vi "Factorial.vi"(1 "N":i32) -> (0 "N!":T1={"Array Num"=[1, 2, 3], "Decimal Index"=0, "stop"=FALSE})   [LabVIEW 2025]
uses:
  Number.ctl
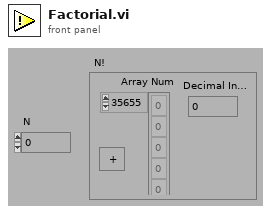
[diagram p1: front panel]
types:
  T1 = typedef "Number.ctl" = cluster{"Array Num":i8[], "Decimal Index":i32, "stop":bool}
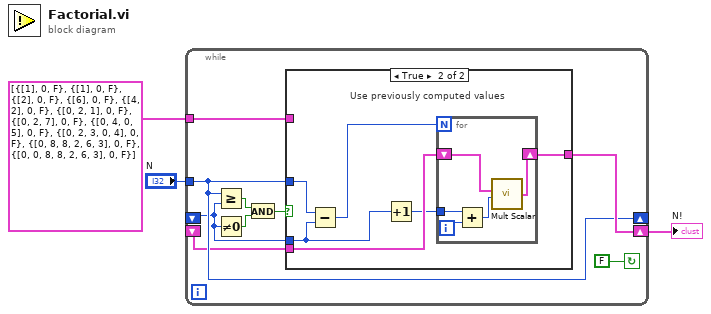
[diagram p0: block diagram]
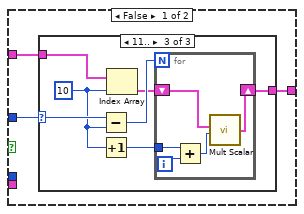
[diagram p2: hidden frame]
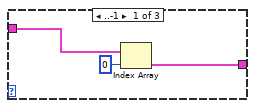
[diagram p3: hidden frame]
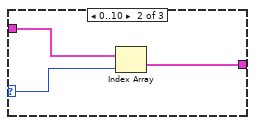
[diagram p4: hidden frame]
diagram:
  n1 = while {
    tunnel: "N" -> [w9]
    tunnel: T1[] [{"Array Num"=[1], "Decimal Index"=0, "stop"=FALSE}, {"Array Num"=[1], "Decimal Index"=0, "stop"=FALSE}, {"Array Num"=[2], "Decimal Index"=0, "stop"=FALSE}, {"Array Num"=[6], "Decimal Index"=0, "stop"=FALSE}, {"Array Num"=[4, 2], "Decimal Index"=0, "stop"=FALSE}, {"Array Num"=[0, 2, 1], "Decimal Index"=0, "stop"=FALSE}, {"Array Num"=[0, 2, 7], "Decimal Index"=0, "stop"=FALSE}, {"Array Num"=[0, 4, 0, 5], "Decimal Index"=0, "stop"=FALSE}, {"Array Num"=[0, 2, 3, 0, 4], "Decimal Index"=0, "stop"=FALSE}, {"Array Num"=[0, 8, 8, 2, 6, 3], "Decimal Index"=0, "stop"=FALSE}, {"Array Num"=[0, 0, 8, 8, 2, 6, 3], "Decimal Index"=0, "stop"=FALSE}] -> [w12]
    shift-right: [w9] -> _
    shift-left: _ -> [w7]
    shift-right: [w10] -> w1
    shift-left: _ -> [w8]
    stop <- FALSE continue-if-true
    n2 = Greater Or Equal?(x=w9, y=w7) -> (x >= y?=w5:bool)
    n3 = Not Equal To 0?(x=w7) -> (x != 0?=w4:bool)
    n4 = And(x=w5, y=w4) -> (x .and. y?=w6:bool)
    n5 = case shown="True" w6 {
      tunnel: w12 -> [w15 _]
      tunnel: [w14 w38] -> w10
      tunnel: w9 -> [w13 w37]
      tunnel: w8 -> [_ w39]
      tunnel: w7 -> [_ w35]
      frame False {
        n6 = case shown="11.." w13 {
          selector: w13 -> [_ w20 w28]
          tunnel: w15 -> [w18 w21 w26]
          tunnel: [w16 w19 w22] -> w14
          frame ..-1 {
            n7 = Index Array(array=w18, index=0) -> (element=w16:T1)
          }
          frame 0..10 {
            n8 = Index Array(array=w21, index=w20) -> (element=w19:T1)
          }
          frame 11.. {
            w24 = 10 ("index")
            n9 = Subtract(x=w28, y=w24) -> (x-y=w27:i32)
            n10 = Increment(x=w24) -> (x+1=w23:i32)
            n11 = Index Array(array=w26, index=w24) -> (element=w25:T1)
            n12 = for {
              N: w27 -> [_]
              tunnel: w23 -> [w33]
              shift-right: [w31] -> w22
              shift-left: w25 -> [w30]
              i -> [w32]
              n13 = Add(x=w33, y=w32) -> (x+y=w29:i32)
              n14 = call "Mult Scalar.vi"("A"=w30, "Scalar"=w29) -> ("A x Scalar"=w31:T1)  [unwired: 3 in]
            }
          }
        }
      }
      frame True {
        # "Use previously computed values"
        n15 = Subtract(x=w37, y=w35) -> (x-y=w36:i32)
        n16 = Increment(x=w35) -> (x+1=w34:i32)
        n17 = for {
          N: w36 -> [_]
          tunnel: w34 -> [w44]
          shift-right: [w42] -> w38
          shift-left: w39 -> [w41]
          i -> [w43]
          n18 = Add(x=w44, y=w43) -> (x+y=w40:i32)
          n19 = call "Mult Scalar.vi"("A"=w41, "Scalar"=w40) -> ("A x Scalar"=w42:T1)  [unwired: 3 in]
        }
      }
    }
  }
  "N!" <- w1
